vi "display.vi"(8 "error in (no error)":errorcluster, 11 "Observer in":refnum<class "Observer.lvclass">) -> (0 "error out":errorcluster, 3 "Observer out":refnum<class "Observer.lvclass">)   [LabVIEW 2020, in "Observer.lvclass"]
uses:
  Observer.lvclass
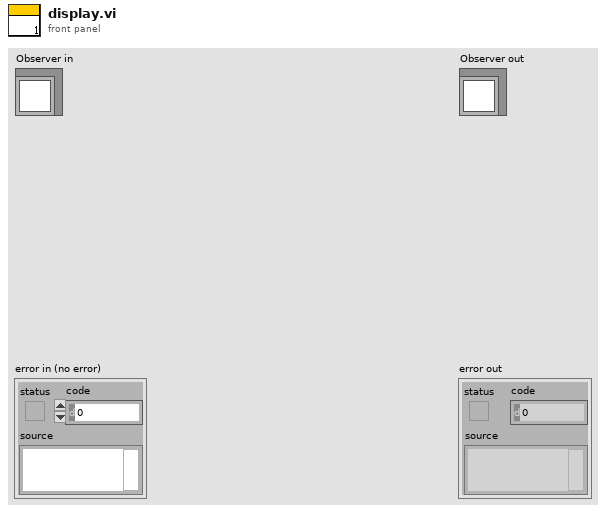
[diagram p1: front panel]
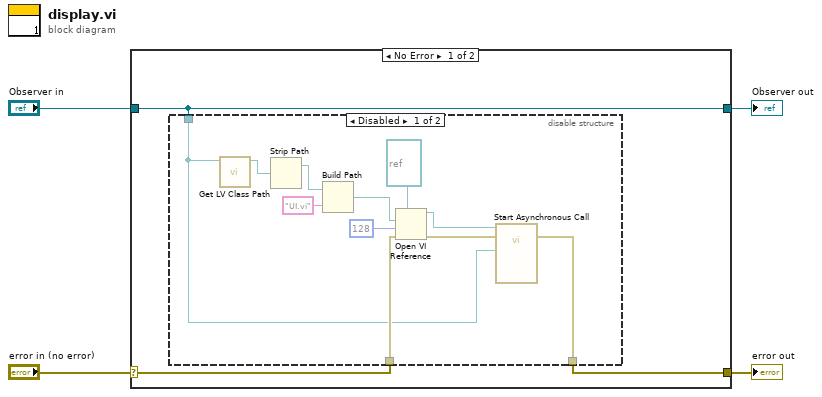
[diagram p0: block diagram]
diagram:
  n1 = case shown="No Error" "error in (no error)" {
    selector: "error in (no error)" -> [w7 w20]
    tunnel: [w6 w20] -> w3
    tunnel: [w5 w19] -> w1
    tunnel: "Observer in" -> [w5 w19]
    frame No Error {
      n2 = disable-structure shown="Disabled" {
        disable-tunnel: w7 -> [w10 _]
        disable-tunnel: [w9 _] -> w6
        disable-tunnel: w5 -> [w8 _]
        frame Disabled {
          n3 = call <vilib>:"Get LV Class Path.vi"("object"=w8) -> ("class path"=w18:path)  [unwired: 9 in, 1 out]
          n4 = Strip Path(path=w18) -> (stripped path=w11:path)  [unwired: 1 out]
          n5 = Build Path(base path=w11, name or relative path="UI.vi") -> (appended path=w16:path)
          n6 = Open VI Reference(type specifier VI Refnum (for type only)=refnum<vi> refnum, vi path=w16, options=128, error in (no error)=w10) -> (vi reference=w14:refnum<vi>, error out=w13:errorcluster)  [unwired: 2 in]
          n7 = call-by-ref "Start Asynchronous Call"(reference=w14, error in=w13, "Observer in"=w8) -> (error out=w9:errorcluster)  [unwired: 9 in, 3 out]
        }
        frame Enabled {
        }
      }
    }
    frame Error {
    }
  }
  "error out" <- w3
  "Observer out" <- w1
